vi "test Parse Sorted Object Dictionary_5.vi"(11 "Test Case In":refnum<class "test Electronic Datasheet.lvclass">) -> (0 "error out":errorcluster, 3 "Test Case Out":refnum<class "test Electronic Datasheet.lvclass">)   [LabVIEW 2024, in "test Electronic Datasheet.lvclass"]
uses:
  test Electronic Datasheet.lvclass
  C:/Program Files/National Instruments/LabVIEW 2024/vi.lib/Astemes/LUnit/Test Case.lvclass
  <vilib>/Astemes/LUnit/Test Case.lvclass/Test Case.ctl
  997a5cc8-28e7-4c8b-bc0c-c7deaea17f55.vi
  <vilib>/Astemes/LUnit/Append Pass Result.vi
  <vilib>/Astemes/LUnit/Append Fail Result.vi
  <vilib>/Astemes/LUnit/Describe Comparison.vi
  997a5cc8-28e7-4c8b-bc0c-c7deaea17f55.vi/9c5d11cd-9439-4240-a1ee-d9baace9c924.vi
  <vilib>/Astemes/LUnit/Run In UI.vi
  <vilib>/Utility/error.llb/Clear Errors.vi
  Electronic Datasheet/utils/Electronic Datasheet_GetAttributes.vi
  <vilib>/Astemes/LUnit/Describe Variant.vi
  Electronic Datasheet/Electronic Datasheet.lvclass
  Core/OD Entry/OD Entry.lvclass
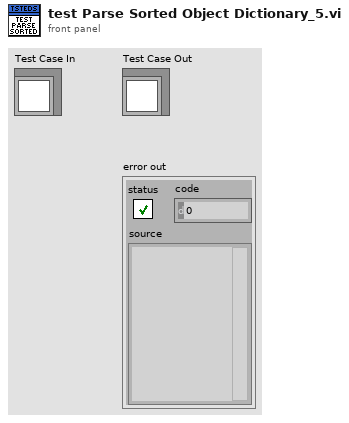
[diagram p1: front panel]
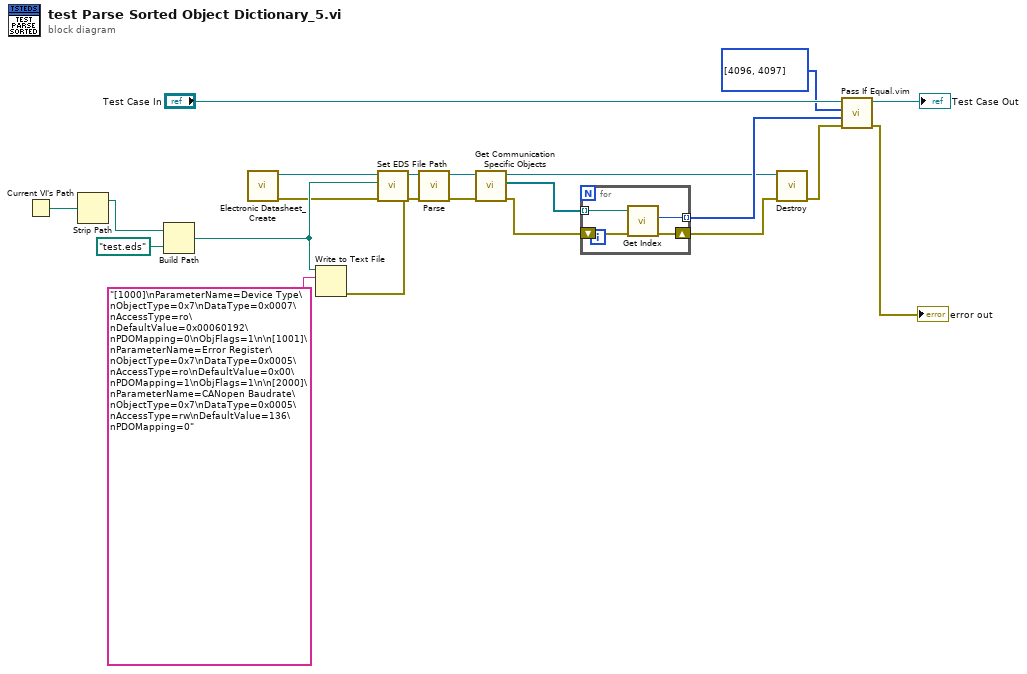
[diagram p0: block diagram]
diagram:
  n1 = Current VI's Path() -> (path=w17:path)
  n2 = Strip Path(path=w17) -> (stripped path=w13:path)  [unwired: 1 out]
  n3 = Build Path(base path=w13, name or relative path=path "test.eds") -> (appended path=w14:path)
  n4 = call "Electronic Datasheet_Create.vi"() -> ("Error Out"=w1:errorcluster, "reference out"=w2:refnum<class "Electronic Datasheet.lvclass">)  [unwired: 10 in]
  n5 = Write to Text File(file (use dialog)=w14, text="[1000]\nParameterName=Device Type\nObjectType=0x7\nDataType=0x0007\nAccessType=ro\nDefaultValue=0x00060192\nPDOMapping=0\nObjFlags=1\n\n[1001]\nParameterName=Error Register\nObjectType=0x7\nDataType=0x0005\nAccessType=ro\nDefaultValue=0x00\nPDOMapping=1\nObjFlags=1\n\n[2000]\nParameterName=CANopen Baudrate\nObjectType=0x7\nDataType=0x0005\nAccessType=rw\nDefaultValue=136\nPDOMapping=0") -> (error out=w15:errorcluster)  [unwired: 2 in, 2 out]
  n6 = call "Set EDS File Path.vi"("error in"=w1, "EDS File Path"=w14, "reference in"=w2) -> ("reference out"=w18:refnum<class "Electronic Datasheet.lvclass">)  [unwired: 7 in, 1 out]
  n7 = call "Parse.vi"("error in"=w15, "reference in"=w18) -> ("error out"=w10:errorcluster, "reference out"=w6:refnum<class "Electronic Datasheet.lvclass">)  [unwired: 8 in]
  n8 = call "Get Communication Specific Objects.vi"("error in"=w10, "Electronic Datasheet"=w6) -> ("error out"=w4:errorcluster, "Entries"=w9:refnum<class "OD Entry.lvclass">[], "Electronic Datasheet"=w5:refnum<class "Electronic Datasheet.lvclass">)  [unwired: 7 in]
  n9 = for {
    tunnel: w9 -> [w25] mode=indexing
    tunnel: [w24] -> w7 mode=indexing
    shift-right: [w22] -> w3
    shift-left: w4 -> [w23]
    n10 = call "Get Index.vi"("Error In"=w23, "reference in"=w25) -> ("Error Out"=w22:errorcluster, "Index"=w24:u16)  [unwired: 7 in, 1 out]
  }
  n11 = call-dynamic "Destroy.vi"("Error In"=w3, "reference in"=w5) -> ("Error Out"=w11:errorcluster)  [unwired: 8 in, 1 out]
  n12 = call "Pass If Equal.vim"("error in (no error)"=w11, "Actual"=w7, "Expected"=u16[] [4096, 4097] ("Array"), "LUnit Test Case In"="Test Case In") -> ("error out"=→"error out":errorcluster, "LUnit Test Case Out"=→"Test Case Out":refnum<class "test Electronic Datasheet.lvclass">)  [unwired: 6 in]
